vi "WPI_MotorControlOpenCANJaguar.vi"(6 "Invert":bool, 8 "error in (no error)":errorcluster, 10 "Device Number":u8, 11 "Control Mode":T5) -> (0 "error out":errorcluster, 3 "MotorControlDeviceRef":T1={"DeviceStatus"={"status"=FALSE, "code"=0, "source"=""}, "Type"=enum."PWM", "PWM"={"PWM Channel"=enum."Invalid", "DeadBand"={"Name"="", "maxPositivePwm"=0, "minPositivePwm"=0, "centerPwm"=0, "maxNegativePwm"=0, "minNegativePwm"=0, "angularRange"=0}}, "CAN"={"Device Number"=0, "SetOutput VI Ref"=variant(enum8{"Percent VBus", "Current", "Speed", "Position", "Voltage"} enum."Percent VBus"), "GetOutput VI Ref"=variant(refnum<k1> refnum), "Enable VI Ref"=variant(dbl 12.0), "Disable VI Ref"=variant(enum8{"Percent VBus", "Speed", "Position", "Slave", "Unchanged / Invalid", "Voltage Compensation", "Current", "Motion Profile"} enum."Percent VBus"), "Data"=variant}, "Invert"=FALSE})   [LabVIEW 2016]
doc: "Creates a reference to the CAN Jaguar motor controller you specify. You must open a reference before using any other VIs on this palette. After you open a reference to the CAN Jaguar motor controller, you can use the SetOutput and GetOutput VIs to set and get the output of the motor controller, respectively.\n\nWhen using closed loop control, you must open the motor controller, configure needed settings (such as PID constants), and then <B>Enable</B> the motor controller.\n\nThis software is licensed. Open the labview\\readme\\WPI Robotics Library Open Source License.txt file for more information."
uses:
  <vilib>/Rock Robotics/WPI/ThirdParty/CanMotor/CAN Jaguar/SubVIs/WPI_CANJaguar_ControlMode.ctl
  <vilib>/Rock Robotics/WPI/MotorControl/WPI_MotorControlDeviceRef.ctl
  <vilib>/Rock Robotics/WPI/MotorControl/WPI_MotorControlType.ctl
  <vilib>/Rock Robotics/SystemInterfaces/DIO/FPGA_DIOPWMChannel.ctl
  <vilib>/Rock Robotics/WPI/PWM/WPI_PWMDeadband.ctl
  <vilib>/Rock Robotics/WPI/ThirdParty/CanMotor/CAN Jaguar/SubVIs/WPI_CANJaguar_RefNumData.ctl
  <vilib>/Rock Robotics/SystemInterfaces/NetworkCommunication/NetComm_UsageReport_ResourceType.ctl
  <vilib>/Rock Robotics/WPI/ThirdParty/CanMotor/CAN Jaguar/SubVIs/WPI_CAN_TokenMessageIDs.ctl
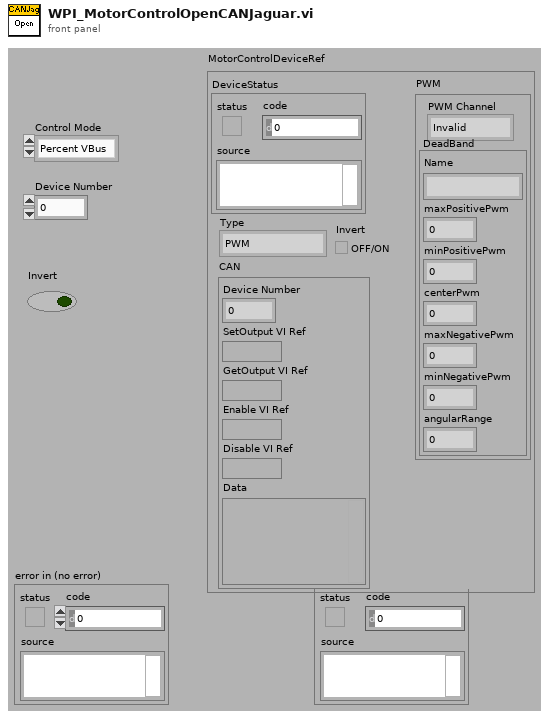
[diagram p1: front panel]
types:
  T1 = typedef "WPI_MotorControlDeviceRef.ctl" = cluster{"DeviceStatus":errorcluster, "Type":T2, "PWM":cluster{"PWM Channel":T3, "DeadBand":T4}, "CAN":cluster{"Device Number":u8, "SetOutput VI Ref":variant, "GetOutput VI Ref":variant, "Enable VI Ref":variant, "Disable VI Ref":variant, "Data":variant}, "Invert":bool}
  T2 = typedef "WPI_MotorControlType.ctl" = enum16{"PWM", "CAN"}
  T3 = typedef "FPGA_DIOPWMChannel.ctl" = enum8{"PWM 0", "PWM 1", "PWM 2", "PWM 3", "PWM 4", "PWM 5", "PWM 6", "PWM 7", "PWM 8", "PWM 9", "PWM MXP 0", "PWM MXP 1", "PWM MXP 2", "PWM MXP 3", "PWM MXP 4", "PWM MXP 5", "PWM MXP 6", "PWM MXP 7", "PWM MXP 8", "PWM MXP 9", "Invalid"}
  T4 = typedef "WPI_PWMDeadband.ctl" = cluster{"Name":string, "maxPositivePwm":i32, "minPositivePwm":i32, "centerPwm":i32, "maxNegativePwm":i32, "minNegativePwm":i32, "angularRange":u16}
  T5 = typedef "WPI_CANJaguar_ControlMode.ctl" = enum8{"Percent VBus", "Current", "Speed", "Position", "Voltage"}
  T6 = typedef "WPI_CANJaguar_RefNumData.ctl" = cluster{"CAN.Max Vout":dbl, "Control Mode":T5, "semaphore":T7}
  T7 = typedef "Semaphore RefNum" = refnum<k1>
  T8 = enum16{"Add", "Remove", "Acquire All", "Release All"}
  T9 = typedef "NetComm_UsageReport_ResourceType.ctl" = enum8{"Controller", "Module", "Language", "CANPlugin", "Accelerometer", "ADXL345", "AnalogChannel", "AnalogTrigger", "AnalogTriggerOutput", "CANJaguar", "Compressor", "Counter", "Dashboard", "DigitalInput", "DigitalOutput", "DriverStationCIO", "DriverStationEIO", "DriverStationLCD", "Encoder", "GearTooth", "Gyro", "I2C", "Framework", "Jaguar", "Joystick", "Kinect", "KinectStick", "PIDController", "Preferences", "PWM", "Relay", "RobotDrive", "SerialPort", "Servo", "Solenoid", "SPI", "Task", "Ultrasonic", "Victor", "Button", "Command", "AxisCamera", "PCVideoServer", "SmartDashboard", "Talon", "HiTechnicColorSensor", "HiTechnicAccel", "HiTechnicCompass", "SRF08", "AnalogOutput", "Victor SP", "Talon SRX", "CAN Talon SRX", "ADXL362 Accel", "ADXRS450 Gyro", "Rev SPARK", "Mindsensors SD540", "Digital Filter"}
  T10 = typedef "WPI_CAN_TokenMessageIDs.ctl" = u32
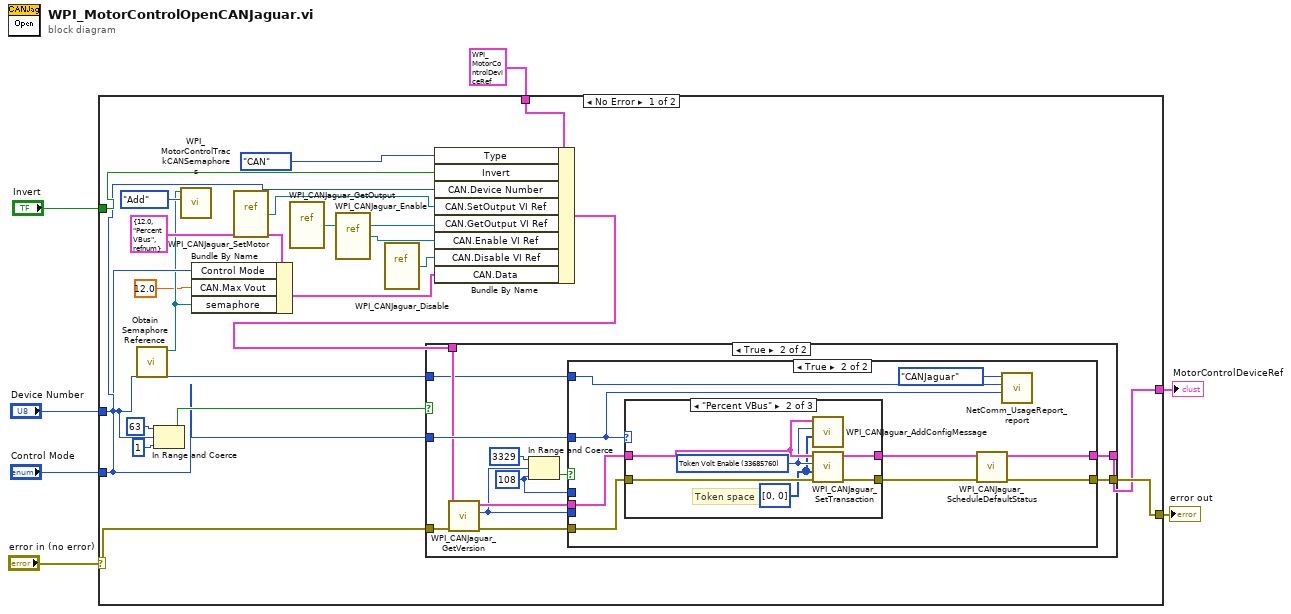
[diagram p0: block diagram]
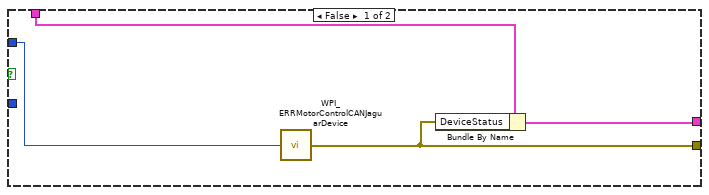
[diagram p2: hidden frame]
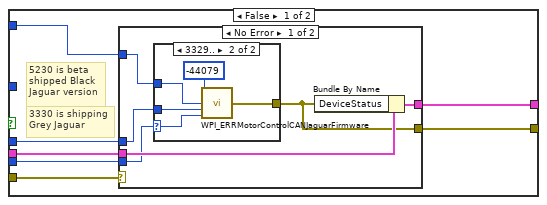
[diagram p3: hidden frame]
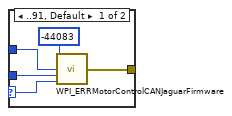
[diagram p4: hidden frame]
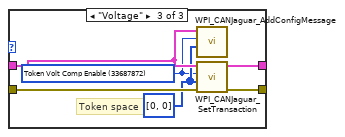
[diagram p7: hidden frame]
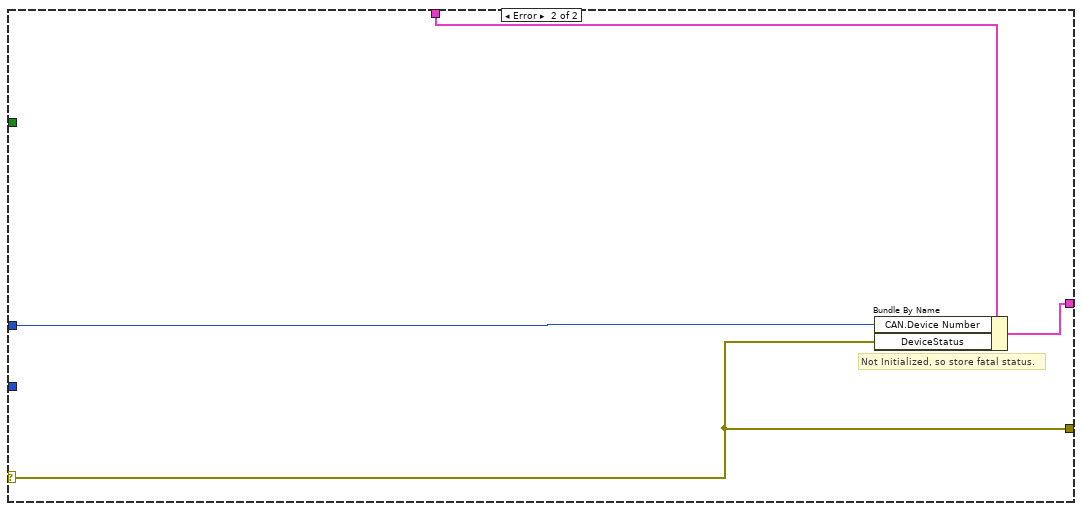
[diagram p8: hidden frame]
diagram:
  n1 = case shown="No Error" "error in (no error)" {
    selector: "error in (no error)" -> [w27 w93]
    tunnel: T1 {"DeviceStatus"={"status"=FALSE, "code"=0, "source"=""}, "Type"=enum."PWM", "PWM"={"PWM Channel"=enum."PWM 1", "DeadBand"={"Name"="", "maxPositivePwm"=0, "minPositivePwm"=0, "centerPwm"=0, "maxNegativePwm"=0, "minNegativePwm"=0, "angularRange"=0}}, "CAN"={"Device Number"=0, "SetOutput VI Ref"=variant(enum8{"Percent VBus", "Current", "Speed", "Position", "Voltage"} enum."Percent VBus"), "GetOutput VI Ref"=variant(refnum<k1> refnum), "Enable VI Ref"=variant(dbl 0.0), "Disable VI Ref"=variant(enum8{"Percent VBus", "Speed", "Position", "Slave", "Unchanged / Invalid", "Voltage Compensation", "Current", "Motion Profile"} enum."Percent VBus"), "Data"=variant}, "Invert"=FALSE} ("CAN Jaguar Ref Out") -> [w28 w96]
    tunnel: [w19 w95] -> w6
    tunnel: [w22 w93] -> w5
    tunnel: "Control Mode" -> [w16 _]
    tunnel: "Device Number" -> [w18 w94]
    tunnel: "Invert" -> [w23 _]
    frame No Error {
      n2 = call <vilib>:"Obtain Semaphore Reference.vi"() -> ("semaphore"=w13:T7)  [unwired: 3 in, 4 out]
      n3 = In Range and Coerce(upper limit=u8 63, x=w18, lower limit=u8 1) -> (In Range?=w24:bool)  [unwired: 1 out]
      n4 = call <vilib>:"WPI_MotorControlTrackCANSemaphores.vi"("Operation"=T8."Add", "semaphore"=w13) -> ()  [unwired: 9 in, 1 out]
      n5 = Bundle By Name(cluster=T6 {"CAN.Max Vout"=12.0, "Control Mode"=enum."Percent VBus", "semaphore"=refnum} ("input cluster"), "Control Mode"=w16, "CAN.Max Vout"=12.0, "semaphore"=w13) -> (w15:T6)
      n6 = vi-ref <vilib>:"WPI_CANJaguar_SetMotor.vi"() -> (w8:refnum<vi>)
      n7 = vi-ref <vilib>:"WPI_CANJaguar_GetOutput.vi"() -> (w11:refnum<vi>)
      n8 = vi-ref <vilib>:"WPI_CANJaguar_Enable.vi"() -> (w10:refnum<vi>)
      n9 = vi-ref <vilib>:"WPI_CANJaguar_Disable.vi"() -> (w9:refnum<vi>)
      n10 = Bundle By Name(cluster=w28, "Type"=WPI_MotorControlType."CAN", "Invert"=w23, "CAN.Device Number"=w18, "CAN.SetOutput VI Ref"=w8, "CAN.GetOutput VI Ref"=w11, "CAN.Enable VI Ref"=w10, "CAN.Disable VI Ref"=w9, "CAN.Data"=w15) -> (w20:T1)
      n11 = case shown="True" w24 {
        tunnel: [w30 w44] -> w22
        tunnel: w16 -> [_ w43]
        tunnel: w18 -> [w29 w34]
        tunnel: w27 -> [_ w42]
        tunnel: w20 -> [w32 w38]
        tunnel: [w31 w36] -> w19
        frame False {
          n12 = call <vilib>:"WPI_ERRMotorControlCANJaguarDevice.vi"("Device Number"=w29) -> ("error out"=w30:errorcluster)  [unwired: 14 out]
          n13 = Bundle By Name(cluster=w32, "DeviceStatus"=w30) -> (w31:T1)
        }
        frame True {
          w33 = u32 108 ("lower limit")
          n14 = call <vilib>:"WPI_CANJaguar_GetVersion.vi"("error in (no error)"=w42, "CAN Jaguar Ref"=w38) -> ("error out"=w41:errorcluster, "Firmware Version"=w35:u32, "CAN Jaguar Ref Out"=w37:T1)  [unwired: 7 out]
          n15 = In Range and Coerce(upper limit=u32 3329, x=w35, lower limit=w33) -> (In Range?=w40:bool)  [unwired: 1 out]
          n16 = case shown="True" w40 {
            tunnel: [w51 w70] -> w44
            tunnel: w43 -> [_ w74]
            tunnel: w41 -> [w50 w77]
            tunnel: w37 -> [w48 w78]
            tunnel: [w49 w71] -> w36
            tunnel: w35 -> [w47 _]
            tunnel: w34 -> [w46 w75]
            tunnel: w33 -> [w45 _]
            frame False {
              # "5230 is beta\nshipped Black\nJaguar version"
              # "3330 is shipping\nGrey Jaguar"
              n17 = case shown="No Error" w50 {
                selector: w50 -> [_ w69]
                tunnel: [w55 w69] -> w51
                tunnel: [w56 w68] -> w49
                tunnel: w48 -> [w57 w68]
                tunnel: w47 -> [w54 _]
                tunnel: w46 -> [w53 _]
                tunnel: w45 -> [w52 _]
                frame No Error {
                  n18 = case shown="3329.." w54 {
                    selector: w54 -> [w61 w66]
                    tunnel: [w62 w67] -> w55
                    tunnel: w53 -> [w60 w65]
                    tunnel: w52 -> [w59 w64]
                    frame ..91, Default {
                      n19 = call <vilib>:"WPI_ERRMotorControlCANJaguarFirmware.vi"("error code"=-44083 ("code"), "Device Number"=w60, "minimum firmware version"=w59, "current firmware version"=w61) -> ("error out"=w62:errorcluster)  [unwired: 11 out]
                    }
                    frame 3329.. {
                      n20 = call <vilib>:"WPI_ERRMotorControlCANJaguarFirmware.vi"("error code"=-44079 ("code"), "Device Number"=w65, "minimum firmware version"=w64, "current firmware version"=w66) -> ("error out"=w67:errorcluster)  [unwired: 11 out]
                    }
                  }
                  n21 = Bundle By Name(cluster=w57, "DeviceStatus"=w55) -> (w56:T1)
                }
                frame Error {
                }
              }
            }
            frame True {
              n22 = case shown="\"Percent VBus\"" w74 {
                tunnel: [w80 w86 w92] -> w72
                tunnel: w77 -> [w80 w85 w91]
                tunnel: w78 -> [w79 w83 w89]
                tunnel: [w79 w84 w90] -> w73
                frame Default {
                }
                frame "Percent VBus" {
                  w82 = T10 33685760 items=["Token Volt Enable"=33685760, "Token Volt Set"=33685824, "Token Volt Set No Ack"=33685952, "Token Speed Enable"=33686976, "Token Speed Set"=33687040, "Token Speed Set No Ack"=33687168, "Token Volt Comp Enable"=33687872, "Token Volt Comp Set"=33687936, "Token Volt Comp Set No Ack"=33688064, "Token Position Enable"=33689024, "Token Position Set"=33689088, "Token Position Set No Ack"=33689216, "Token Current Enable"=33689984, "Token Current Set"=33690048, "Token Current Set No Ack"=33690176] ("CAN Token Message IDs")
                  w81 = u8[] [0, 0] ("data")
                  # "Token space"
                  n23 = call <vilib>:"WPI_CANJaguar_AddConfigMessage.vi"("Data"=w81, "Message ID"=w82, "CAN Jaguar Ref"=w83) -> ()  [unwired: 9 in]
                  n24 = call <vilib>:"WPI_CANJaguar_SetTransaction.vi"("error in"=w85, "Data"=w81, "Message ID"=w82, "CAN Jaguar Ref"=w83) -> ("error out"=w86:errorcluster, "CAN Jaguar Ref Out"=w84:T1)  [unwired: 6 out]
                }
                frame "Voltage" {
                  w87 = T10 33687872 items=["Token Volt Enable"=33685760, "Token Volt Set"=33685824, "Token Volt Set No Ack"=33685952, "Token Speed Enable"=33686976, "Token Speed Set"=33687040, "Token Speed Set No Ack"=33687168, "Token Volt Comp Enable"=33687872, "Token Volt Comp Set"=33687936, "Token Volt Comp Set No Ack"=33688064, "Token Position Enable"=33689024, "Token Position Set"=33689088, "Token Position Set No Ack"=33689216, "Token Current Enable"=33689984, "Token Current Set"=33690048, "Token Current Set No Ack"=33690176] ("CAN Token Message IDs")
                  w88 = u8[] [0, 0] ("data")
                  # "Token space"
                  n25 = call <vilib>:"WPI_CANJaguar_AddConfigMessage.vi"("Data"=w88, "Message ID"=w87, "CAN Jaguar Ref"=w89) -> ()  [unwired: 9 in]
                  n26 = call <vilib>:"WPI_CANJaguar_SetTransaction.vi"("error in"=w91, "Data"=w88, "Message ID"=w87, "CAN Jaguar Ref"=w89) -> ("error out"=w92:errorcluster, "CAN Jaguar Ref Out"=w90:T1)  [unwired: 6 out]
                }
              }
              n27 = call <vilib>:"WPI_CANJaguar_ScheduleDefaultStatus.vi"("error in (no error)"=w72, "CAN Jaguar Ref Out in"=w73) -> ("error out"=w70:errorcluster, "CAN Jaguar Ref Out out"=w71:T1)  [unwired: 8 in]
              n28 = call <vilib>:"NetComm_UsageReport_report.vi"("Context"=w74, "Instance Number"=w75, "Resource Type"=NetComm_UsageReport_ResourceType."CANJaguar") -> ()  [unwired: 9 in]
            }
          }
        }
      }
    }
    frame Error {
      # "Not Initialized, so store fatal status."
      n29 = Bundle By Name(cluster=w96, "CAN.Device Number"=w94, "DeviceStatus"=w93) -> (w95:T1)
    }
  }
  "error out" <- w5
  "MotorControlDeviceRef" <- w6
